vi "IPCheck.vi"() -> ()   [LabVIEW 2018]
panel:
  out "匹配子字符串":string
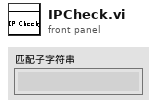
[diagram p1: front panel]
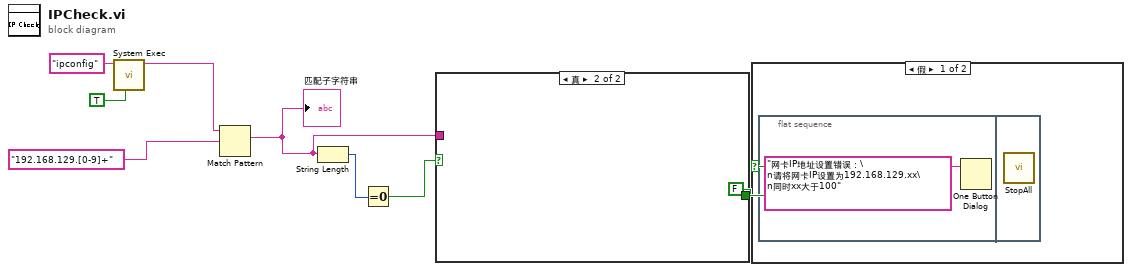
[diagram p0: block diagram]
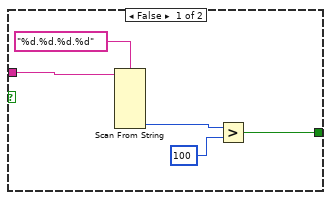
[diagram p3: hidden frame]
diagram:
  n1 = call <vilib>:"System Exec.vi"("run minimized? (F)"=TRUE, "command line"="ipconfig") -> ("standard output"=w7:string)  [unwired: 6 in, 3 out]
  n2 = Match Pattern(string=w7, regular expression="192.168.129.[0-9]+" ("正则表达式")) -> (match substring=w3:string)  [unwired: 1 in, 3 out]
  "匹配子字符串" <- w3
  n3 = String Length(string=w3) -> (length=w5:i32)
  n4 = Equal To 0?(x=w5) -> (x = 0?=w4:bool)
  n5 = case shown="真" w4 {
    tunnel: w3 -> [w13 _]
    tunnel: [w9 FALSE] -> w1
    frame False {
      n6 = Scan From String(format string="%d.%d.%d.%d" ("格式字符串"), input string=w13) -> (output 4=w11:i32)  [unwired: 9 in, 3 out]
      n7 = Greater?(x=w11, y=100) -> (0:w9:bool)
    }
    frame True {
    }
  }
  n8 = case shown="假" w1 {
    frame False {
      n9 = flat-sequence {
        frame #0 {
          n10 = One Button Dialog(message="网卡IP地址设置错误：\n请将网卡IP设置为192.168.129.xx\n同时xx大于100" ("消息")) -> ()  [unwired: 1 in, 1 out]
        }
        frame #1 {
          n11 = call "StopAll.vi"() -> ()  [unwired: 12 in]
        }
      }
    }
    frame True {
    }
  }
